vi "Acquire Data from Hardware.vi"(8 "error in (no error)":errorcluster, 9 "read":bool, 10 "Network":T4={"invert_send"=TRUE, "Number of datagrams to read"=5000, "max bytes/read"=2500, "Timeout"=4000, "host"="192.168.1.18", "Port Receive"=5678} {"Number of datagrams to read" format="%0d"}, 11 "Acquisition Settings":T5) -> (0 "error out":errorcluster, 1 "Graph Data 2":T1, 2 "Graph Data":waveform(dbl)[](array[waveform]))   [LabVIEW 2014]
doc: "Generates sample waveforms according to the signal type in the HW Config input."
uses:
  controls/DAQSettings.ctl
  controls/TriggerMode.ctl
  controls/Network.ctl
  controls/Graph Data.ctl
  <vilib>/Utility/miscctls.llb/LVAnnotationListTypeDef.ctl
  <vilib>/Utility/miscctls.llb/LVCursorListTypeDef.ctl
  controls/CommSelect.ctl
panel:
  out "voidcount 2":dbl
  in  "voidcount":dbl
  out "DATA":string
  out "zhile loop":i32
  out "data out":string
  in  "error in (no error) 2":errorcluster
  in  "stop":bool
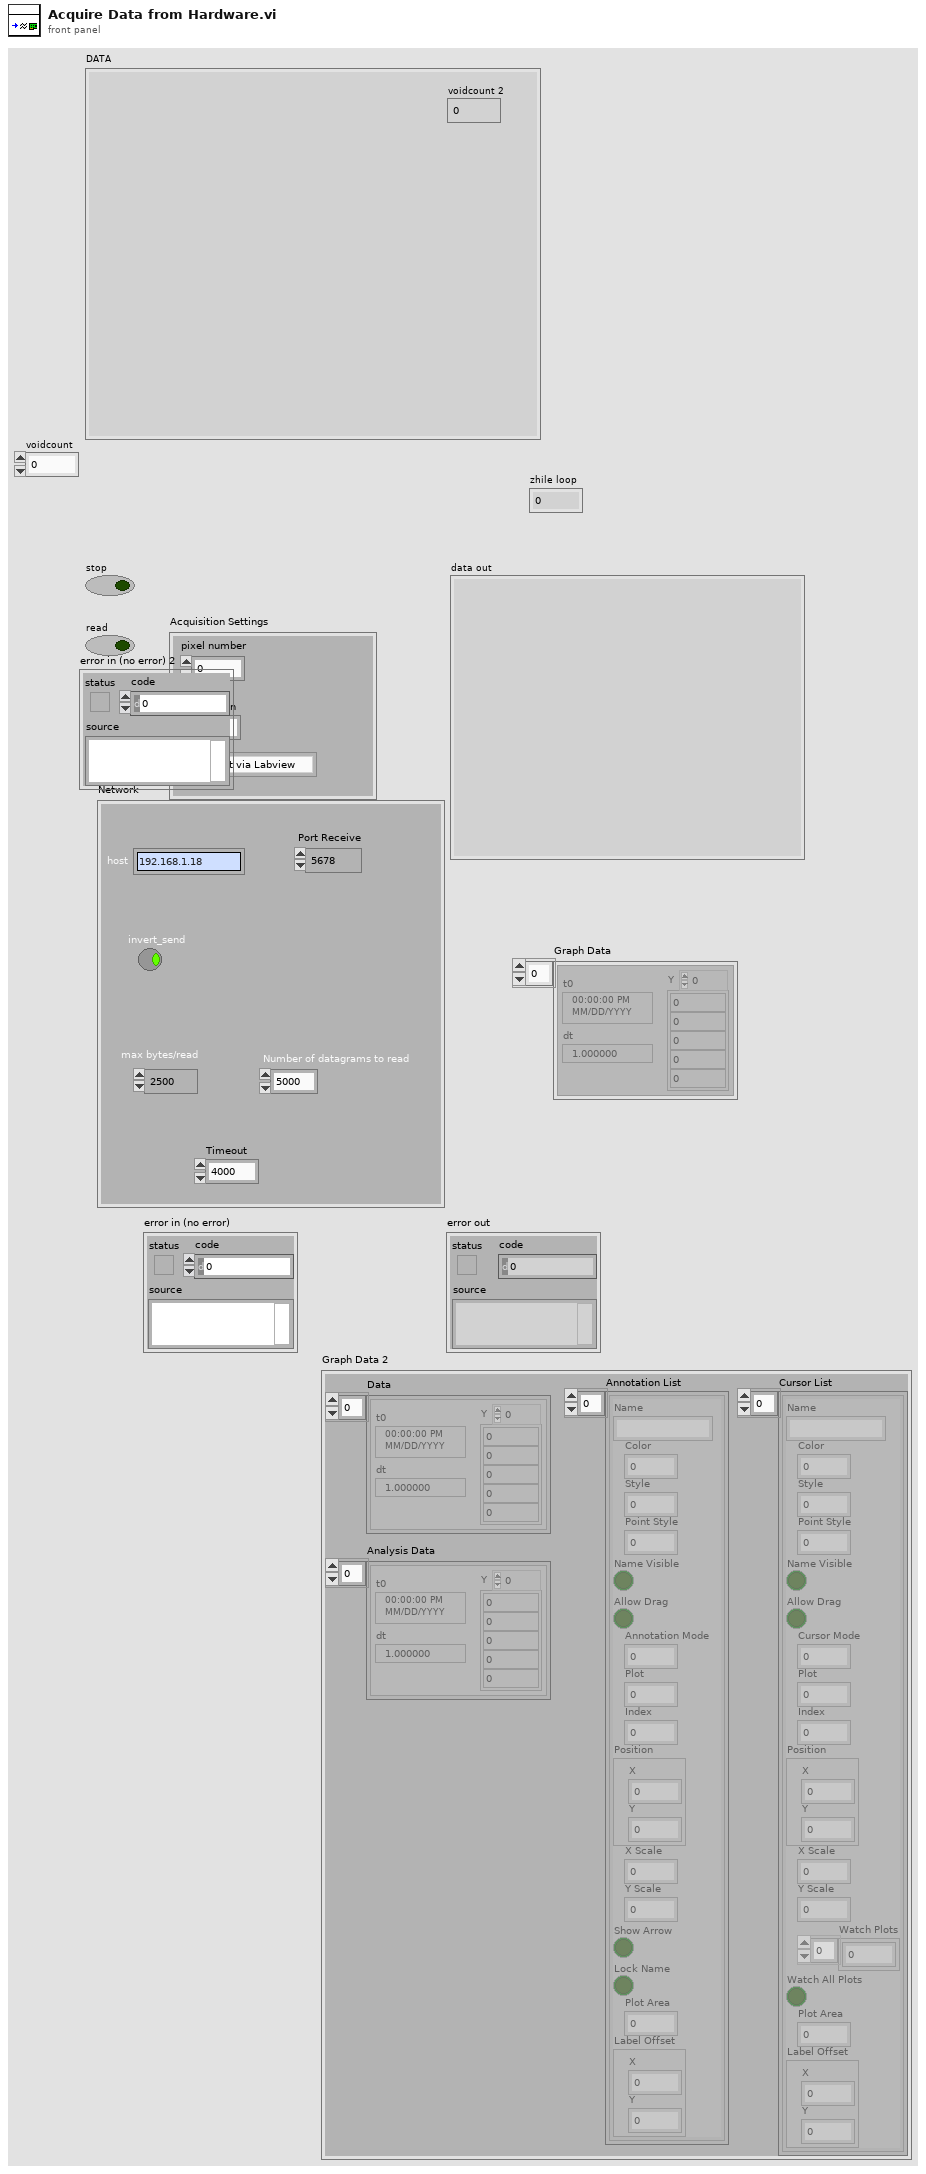
[diagram p1: front panel]
types:
  T1 = typedef "Graph Data.ctl" = cluster{"Data":waveform(dbl)[], "Annotation List":T2, "Cursor List":T3, "Analysis Data":waveform(dbl)[]}
  T2 = typedef "LVAnnotationListTypeDef.ctl" = cluster{"Name":string, "Color":u32, "Style":u8, "Point Style":u8, "Name Visible":bool, "Allow Drag":bool, "Annotation Mode":u32, "Plot":i32, "Index":i32, "Position":cluster{"X":dbl, "Y":dbl}, "X Scale":u32, "Y Scale":u32, "Show Arrow":bool, "Lock Name":bool, "Plot Area":i32, "Label Offset":cluster{"X":dbl, "Y":dbl}}[]
  T3 = typedef "LVCursorListTypeDef.ctl" = cluster{"Name":string, "Color":u32, "Style":u8, "Point Style":u8, "Name Visible":bool, "Allow Drag":bool, "Cursor Mode":u32, "Plot":i32, "Index":i32, "Position":cluster{"X":dbl, "Y":dbl}, "X Scale":u32, "Y Scale":u32, "Watch Plots":i32[], "Watch All Plots":bool, "Plot Area":i32, "Label Offset":cluster{"X":dbl, "Y":dbl}}[]
  T4 = typedef "Network.ctl" = cluster{"invert_send":bool, "Number of datagrams to read":u32, "max bytes/read":i32, "Timeout":i32, "host":string, "Port Receive":u16}
  T5 = typedef "DAQSettings.ctl" = cluster{"pixel number":u32, "repetition":u32, "Trigger":T6}
  T6 = typedef "TriggerMode.ctl" = enum16{"Ethernet via Labview", "SMA (1.8V)"}
  T7 = typedef "CommSelect.ctl" = enum16{"startTSL", "writeCABAC", "readCABAC", "resetCABAC", "emissionTest", "regRead", "executeASPIC", "resetASPIC", "resetFifo18ASPIC", "resetFifo16ASPIC", "LabviewDamicStart"}
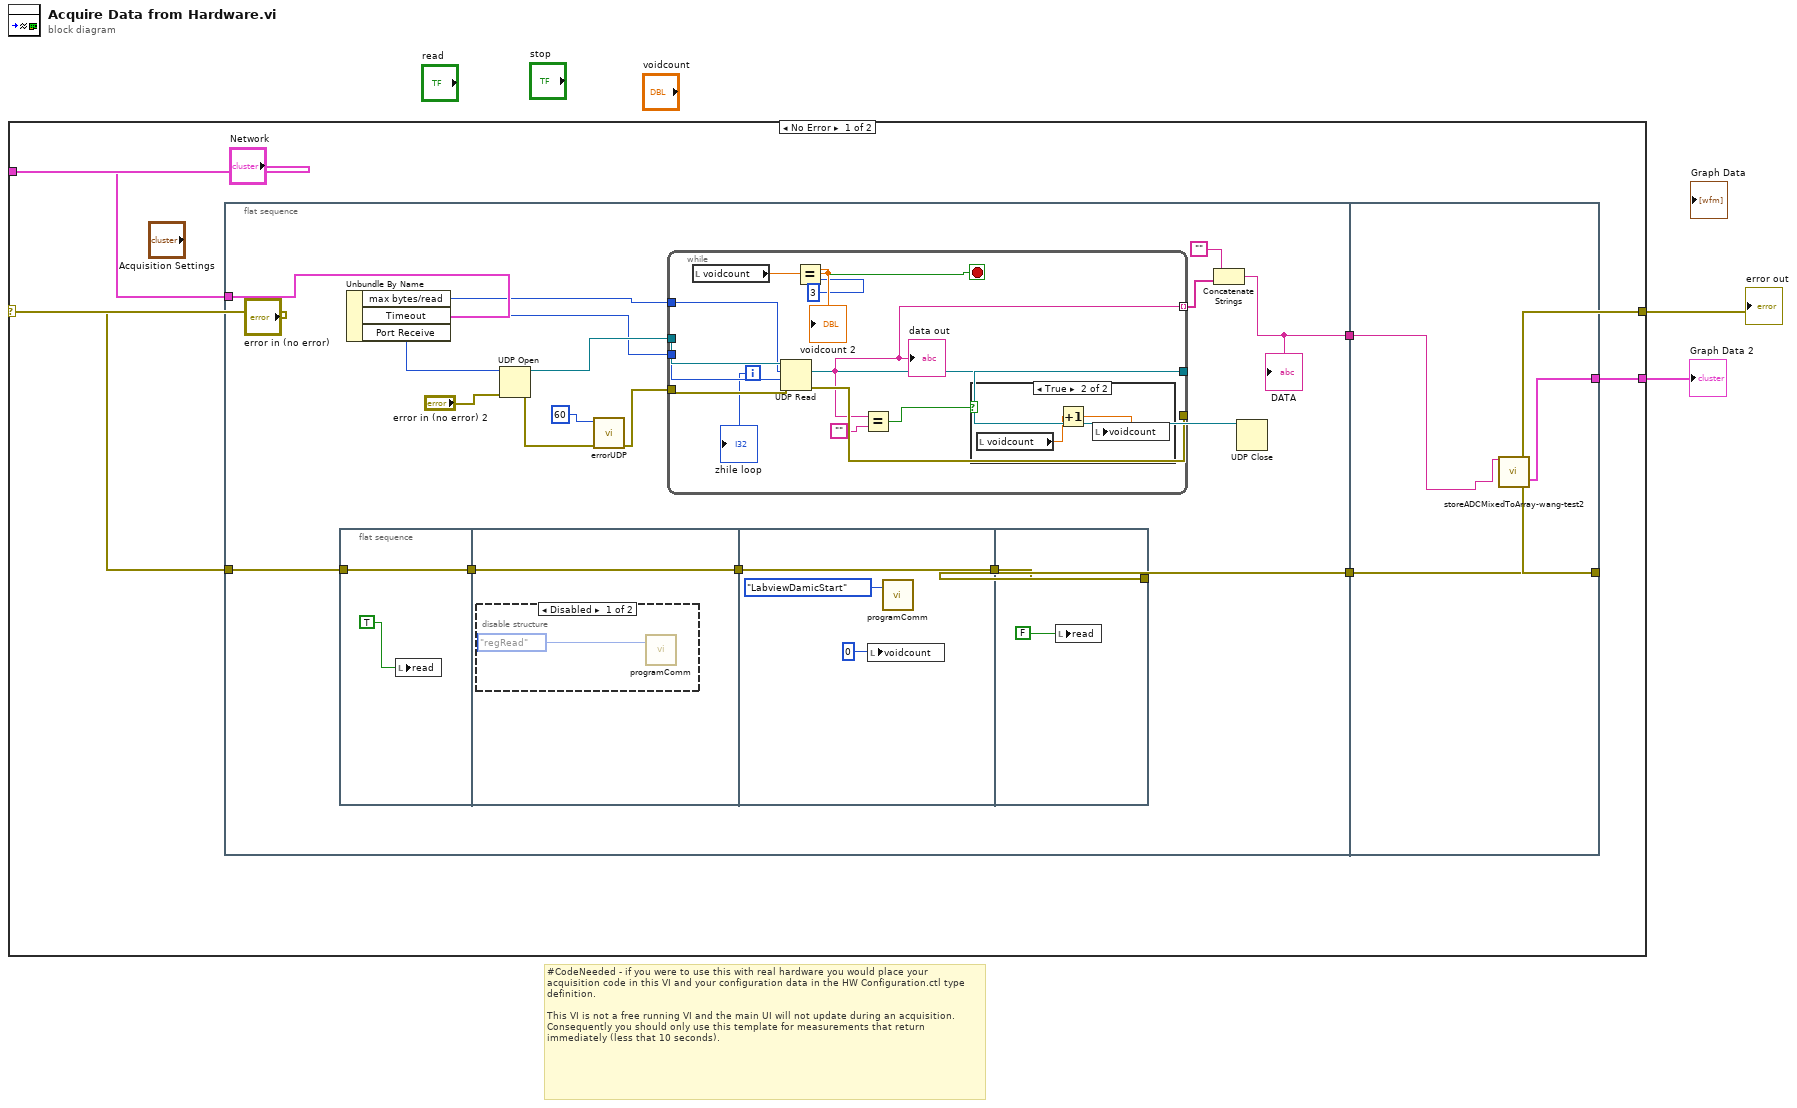
[diagram p0: block diagram]
diagram:
  # "#CodeNeeded - if you were to use this with real hardware you would place your acquisition code in this VI and your configuration data in the HW Configuration.ctl type definition.\n\nThis VI is not a free running VI and the main UI will not update during an acquisition.  Consequently you should only use this template for measurements that return immediately (less that 10 seconds)."
  n1 = case shown="No Error" "error in (no error)" {
    selector: "error in (no error)" -> [w10 w56]
    tunnel: [w6 w56] -> w2
    tunnel: "Network" -> [w9 _]
    tunnel: [w5 _] -> w1
    frame No Error {
      n2 = flat-sequence {
        tunnel: w10 -> [w28]
        tunnel: w9 -> [w27]
        tunnel: [w17] -> w8
        tunnel: [w15] -> w7
        tunnel: w8 -> [w54]
        tunnel: [w55] -> w6
        tunnel: w7 -> [w55]
        tunnel: [w53] -> w5
        frame #0 {
          n3 = flat-sequence {
            tunnel: w28 -> [w44]
            tunnel: [w44] -> w14
            tunnel: w14 -> [w46]
            tunnel: [w46] -> w13
            tunnel: [w48] -> w16
            tunnel: w13 -> [w48]
            tunnel: [w51] -> w15
            tunnel: w16 -> [w51]
            frame #0 {
              n4 = local write "read"(TRUE) -> ()
            }
            frame #1 {
              n5 = disable-structure shown="Disabled" {
                frame Disabled {
                  n6 = call "programComm.vi"("CommSelect"=CommSelect."regRead") -> ()  [unwired: 1 in, 1 out]
                }
                frame Enabled {
                }
              }
            }
            frame #2 {
              n7 = local write "voidcount"(0) -> ()
              n8 = call "programComm.vi"("CommSelect"=CommSelect."LabviewDamicStart") -> ()  [unwired: 1 in, 1 out]
            }
            frame #3 {
              n9 = local write "read"(FALSE) -> ()
            }
          }
          n10 = Unbundle By Name(w27) -> ("max bytes/read"=w23:i32, "Timeout"=w22:i32, "Port Receive"=w25:u16)
          n11 = UDP Open(8:"error in (no error) 2", 11:w25) -> (port=w24:refnum<k16>, 0:w20:errorcluster)  [unwired: 4 out]
          n12 = call "errorUDP.vi"("error in (no error) 2"=w20, "errorcode"=60) -> ("error out 2"=w18:errorcluster)  [unwired: 9 out]
          n13 = while {
            tunnel: w18 -> [w41]
            tunnel: [w40] -> _
            tunnel: w24 -> [w39]
            tunnel: w23 -> [w38]
            tunnel: w22 -> [w37]
            tunnel: [w35] -> w21
            tunnel: [w34] -> w11 mode=indexing
            i -> [w36]
            stop <- w29 stop-if-true
            n14 = local read "voidcount"() -> (w31:dbl)
            "voidcount 2" <- w31
            n15 = UDP Read(connection ID=w39, max size (548)=w38, timeout ms (25000)=w37, 8:w41) -> (data out=w34:string, error out=w40:errorcluster, 3:w35:refnum<k16>)  [unwired: 2 out]
            "data out" <- w34
            n16 = Equal?(x=w31, y=3) -> (x = y?=w29:bool)
            n17 = Equal?(x=w34, y="") -> (x = y?=w32:bool)
            n18 = case shown="True" w32 {
              frame False {
              }
              frame True {
                n19 = local read "voidcount"() -> (w43:dbl)
                n20 = Increment(x=w43) -> (x+1=w42:dbl)
                n21 = local write "voidcount"(w42) -> ()
              }
            }
            "zhile loop" <- w36
          }
          n22 = Concatenate Strings("", w11) -> (w17:string)
          "DATA" <- w17
          n23 = UDP Close(connection ID=w21) -> ()  [unwired: 1 in, 2 out]
        }
        frame #1 {
          n24 = call "storeADCMixedToArray-wang-test2.vi"("String"=w54) -> ("Graph Data"=w53:T1)  [unwired: 17 in, 1 out]
        }
      }
    }
    frame Error {
    }
  }
  "error out" <- w2
  "Graph Data 2" <- w1
